vi "Station Update Instruments.vi"(8 "error in (no error)":errorcluster, 9 "Instruments on Station":T1[](array[typedef]), 10 "Station KEY (0)":i32, 11 "Connection Refnum":T2) -> (0 "error out":errorcluster, 3 "Connection Refnum":T2)   [LabVIEW 2011]
uses:
  SI.LIB/ODBC/SQL Controls/Connection Refnum.ctl
  Instruments/Instrument Record.ctl
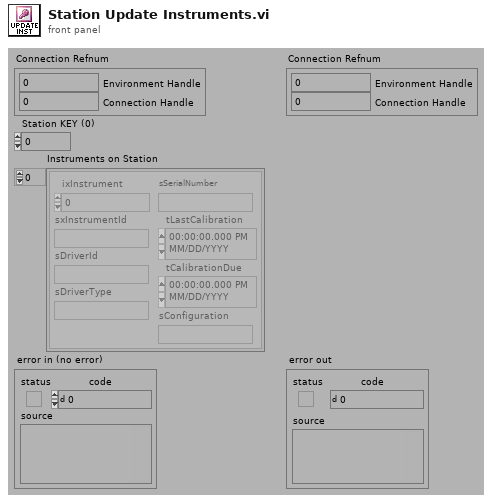
[diagram p1: front panel]
types:
  T1 = typedef "Instrument Record.ctl" = cluster{"ixInstrument":i32, "sxInstrumentId":string, "sDriverId":string, "sDriverType":string, "sSerialNumber":string, "tLastCalibration":timestamp, "tCalibrationDue":timestamp, "sConfiguration":string}
  T2 = typedef "Connection Refnum.ctl" = cluster{"Environment Handle":i32, "Connection Handle":i32}
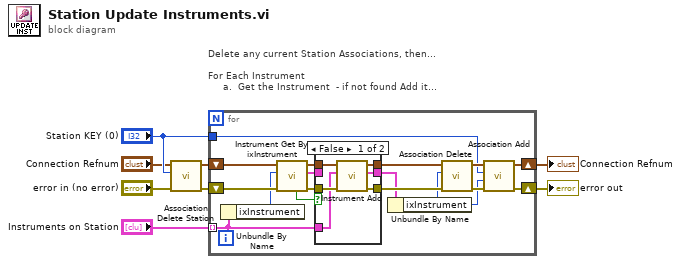
[diagram p0: block diagram]
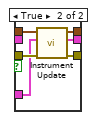
[diagram p2: hidden frame]
diagram:
  n1 = call "Association Delete Station.vi"("error in (no error)"="error in (no error)", "iStation (0)"="Station KEY (0)", "Connection Refnum"="Connection Refnum") -> ("error out"=w6:errorcluster, "Connection Refnum"=w7:T2)  [unwired: 7 out]
  n2 = for "Delete any current Station Associations, then...\n \nFor Each Instrument\n     a.  Get the Instrument  - if not found Add it, if found update it\n     b.  Remove all associations (make Free)\n     c.  Add associations to new Station" {
    tunnel: "Instruments on Station" -> [w19] mode=indexing
    shift-right: [w12] -> w3
    shift-left: w6 -> [w24]
    shift-right: [w13] -> w4
    shift-left: w7 -> [w25]
    tunnel: "Station KEY (0)" -> [w10]
    n3 = Unbundle By Name(w19) -> ("ixInstrument"=w9:i32)
    n4 = call "Instrument Get By ixInstrument.vi"("error in (no error)"=w24, "ixInstrument"=w9, "Connection Refnum"=w25) -> ("error out"=w22:errorcluster, "Instrument Record"=w20:T1, "Connection Refnum"=w21:T2, "Data Present?"=w23:bool)  [unwired: 5 out]
    n5 = case shown="False" w23 {
      tunnel: w22 -> [w30 w36]
      tunnel: w21 -> [w31 w37]
      tunnel: w20 -> [_ _]
      tunnel: [w26 w35] -> w17
      tunnel: [w27 w34] -> w18
      tunnel: [w28 w33] -> w16
      tunnel: w19 -> [w29 w32]
      frame False {
        n6 = call "Instrument Add.vi"("error in (no error)"=w30, "Instrument Record"=w29, "Connection Refnum"=w31) -> ("error out"=w26:errorcluster, "New Instrument Record"=w28:T1, "Connection Refnum"=w27:T2)  [unwired: 6 out]
      }
      frame True {
        n7 = call "Instrument Update.vi"("error in (no error)"=w36, "Instrument Record"=w32, "Connection Refnum"=w37) -> ("error out"=w35:errorcluster, "Updated Instrument"=w33:T1, "Connection Refnum"=w34:T2)  [unwired: 6 out]
      }
    }
    n8 = Unbundle By Name(w16) -> ("ixInstrument"=w11:i32)
    n9 = call "Association Delete.vi"("error in (no error)"=w17, "iInstrument (0)"=w11, "Connection Refnum"=w18) -> ("error out"=w14:errorcluster, "Connection Refnum"=w15:T2)  [unwired: 7 out]
    n10 = call "Association Add.vi"("error in (no error)"=w14, "iInstrument (0)"=w11, "iStation (0)"=w10, "Connection Refnum"=w15) -> ("error out"=w12:errorcluster, "Connection Refnum"=w13:T2)  [unwired: 6 out]
  }
  "error out" <- w3
  "Connection Refnum" <- w4
